vi "MFCCalAssistant.vi"() -> ()   [LabVIEW 2016]
doc: "Use this template to build a simple state machine design pattern. Each state executes code and determines which state to transition to."
uses:
  MFCCallAssistant-State.ctl
  MFCCalAssistant-Data.ctl
  Anemometry Sub Vis/Globals/Preference_global.vi
panel:
  out "Pressure":dbl format="%.1fmBar"
  out "Temp":dbl format="%.1fC"
  out "Gauge":dbl(knob) scale=0.0..10.0
  in  "Cal Gas":string(combo)
  out "Flow Rate (g/min)":dbl
  out "Flow Rate (l/min)":dbl
  out "Metered Gas Volume (ft^3)":dbl
  out "Elapsed Time (s)":dbl format="%.2f"
  out "Timer On":bool caption="(Press spacebar to toggle timer.)"
  in  "Reset Button":bool
  in  "Exit":bool
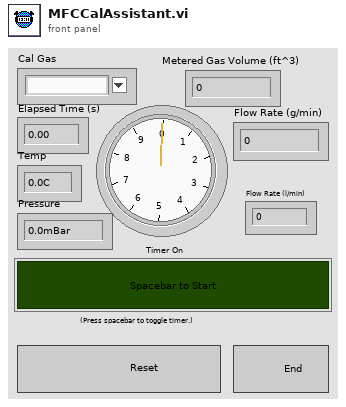
[diagram p1: front panel]
types:
  T1 = typedef "MFCCalAssistant-Data.ctl" = cluster{"Timer on?":bool, "Start Time":dbl, "Stop Time":dbl, "Elapsed Time (s)":dbl, "Measured Gas Volume (ft^3)":dbl, "Converted Gas Volume (l)":dbl, "Flow Rate (l/min)":dbl, "Flow Rate (g/min)":dbl}
  T2 = typedef "MFCCallAssistant-State.ctl" = enum16{"Initialize", "Wait for Event", "Toggle Timer", "Get User Data", "Compute Results", "Display Results", "Exit"}
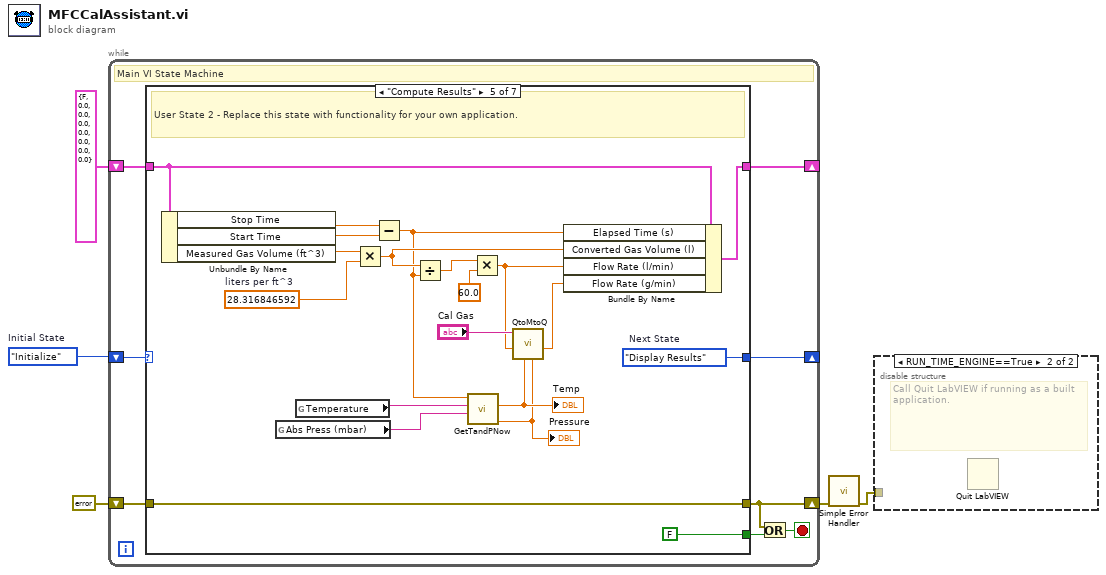
[diagram p0: block diagram]
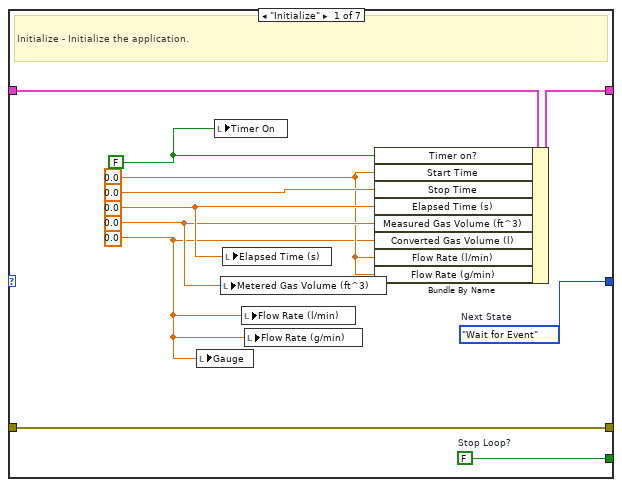
[diagram p3: hidden frame]
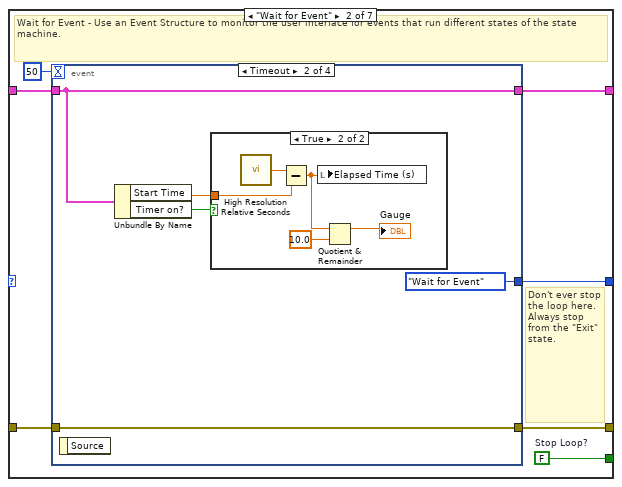
[diagram p4: hidden frame]
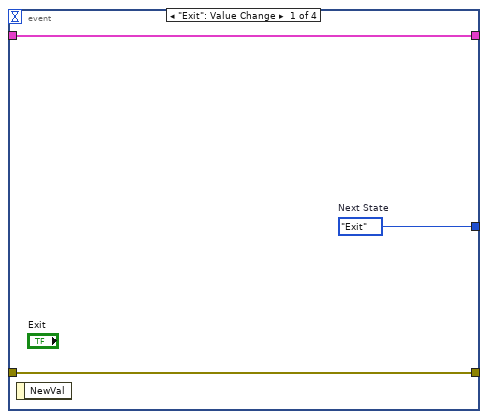
[diagram p5: hidden frame]
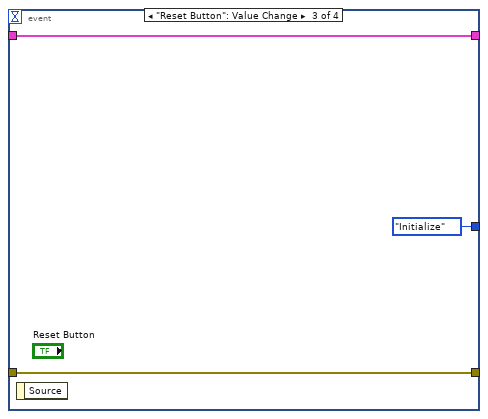
[diagram p7: hidden frame]
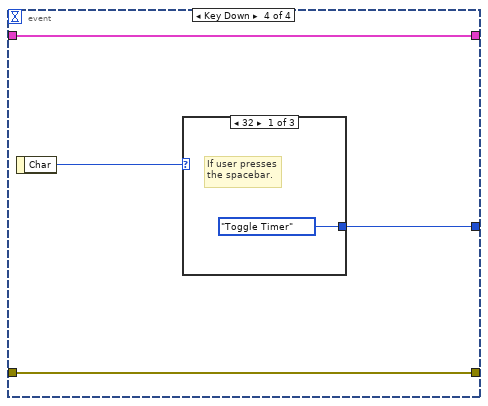
[diagram p8: hidden frame]
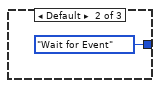
[diagram p9: hidden frame]
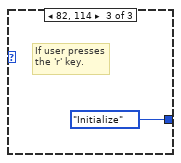
[diagram p10: hidden frame]
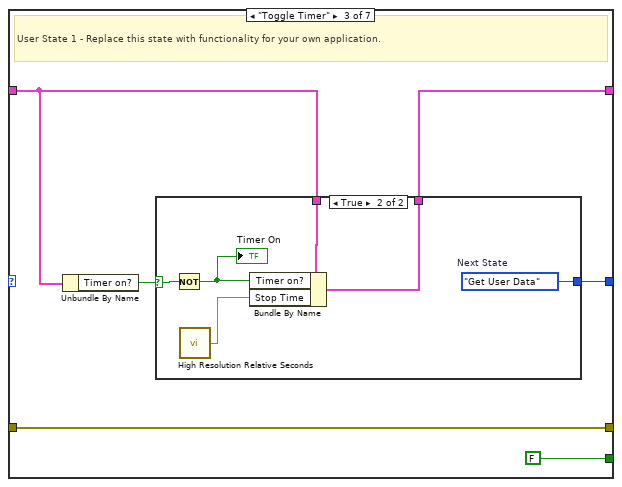
[diagram p11: hidden frame]
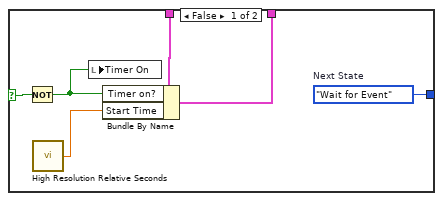
[diagram p12: hidden frame]
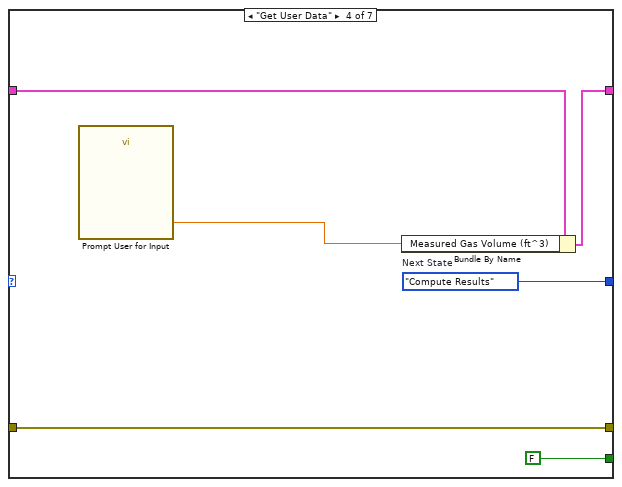
[diagram p13: hidden frame]
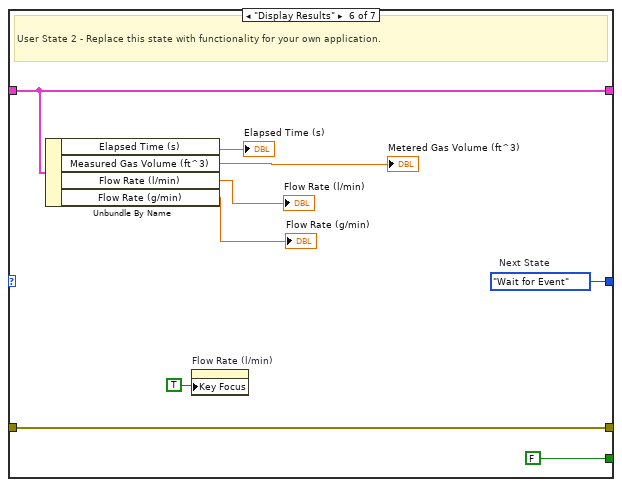
[diagram p14: hidden frame]
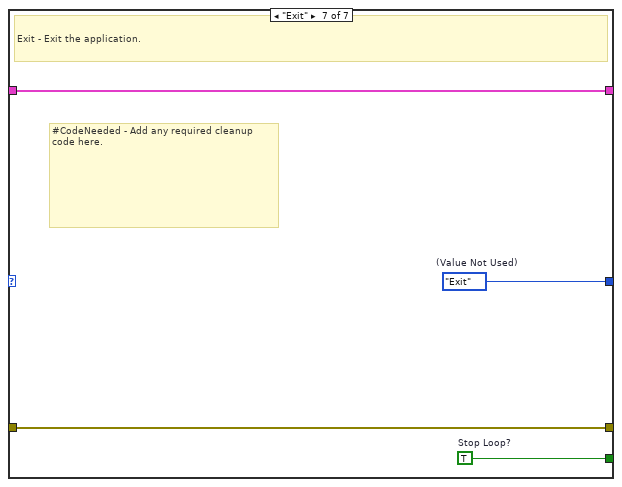
[diagram p15: hidden frame]
diagram:
  w5 = MFCCallAssistant-State."Initialize"  # Initial State
  n1 = while {
    shift-right: [w12] -> _
    shift-left: w5 -> [w13]
    shift-right: [w10] -> _
    shift-left: T1 {"Timer on?"=FALSE, "Start Time"=0.0, "Stop Time"=0.0, "Elapsed Time (s)"=0.0, "Measured Gas Volume (ft^3)"=0.0, "Converted Gas Volume (l)"=0.0, "Flow Rate (l/min)"=0.0, "Flow Rate (g/min)"=0.0} ("Data") -> [w11]
    shift-right: [w6] -> w2
    shift-left: errorcluster {"status"=FALSE, "code"=0, "source"=""} ("error constant") -> [w9]
    stop <- w7 stop-if-true
    # "Main VI State Machine"
    n2 = case shown="\"Compute Results\"" w13 {
      tunnel: [w24 w31 w57 w74 w98 w107 w111] -> w12
      tunnel: [w23 w30 FALSE ("Stop Loop?") FALSE ("Stop Loop?") FALSE ("Stop Loop?") FALSE ("Stop Loop?") w109] -> w8
      tunnel: w11 -> [w22 w29 w56 w77 w94 w104 w110]
      tunnel: [w21 w28 w55 w75 w93 w104 w110] -> w10
      tunnel: w9 -> [w20 w27 w59 w78 w96 w105 w108]
      tunnel: [w20 w26 w59 w78 w96 w105 w108] -> w6
      frame "Initialize" {
        w14 = 0.0 ("Converted Gas Volume")
        w16 = 0.0 ("Integrated Gas Volume")
        w17 = 0.0 ("Elapsed Time")
        w15 = 0.0 ("Stop Time")
        w18 = FALSE ("Replace_Me_Boolean")
        w23 = FALSE  # Stop Loop?
        w24 = MFCCallAssistant-State."Wait for Event"  # Next State
        # "Initialize - Initialize the application."
        n3 = local write "Gauge"(w14) -> ()
        n4 = local write "Timer On"(w18) -> ()
        n5 = local write "Metered Gas Volume (ft^3)"(w16) -> ()
        n6 = local write "Elapsed Time (s)"(w17) -> ()
        n7 = local write "Flow Rate (l/min)"(w14) -> ()
        n8 = local write "Flow Rate (g/min)"(w14) -> ()
        n9 = Bundle By Name(cluster=w22, "Timer on?"=w18, "Start Time"=w15, "Stop Time"=0.0 ("Start Time"), "Elapsed Time (s)"=w17, "Measured Gas Volume (ft^3)"=w16, "Converted Gas Volume (l)"=w14, "Flow Rate (l/min)"=w15, "Flow Rate (g/min)"=w15) -> (w21:T1)
      }
      frame "Wait for Event" {
        w30 = FALSE  # Stop Loop?
        # "Don't ever stop the loop here. Always stop from the \"Exit\" state."
        # "Wait for Event - Use an Event Structure to monitor the user interface for events that run different states of the state machine."
        n10 = event shown="[1] Timeout" {
          selector: _ -> [_ _ _ _]
          dyn-events: _ -> [_ _ _ _]
          timeout: 50 -> [_ _ _ _]
          tunnel: [w34 MFCCallAssistant-State."Wait for Event" ("Next State") MFCCallAssistant-State."Initialize" ("Next State") w48] -> w31
          tunnel: w29 -> [w33 w36 w47 w51]
          tunnel: [w33 w36 w47 w51] -> w28
          tunnel: w27 -> [w32 w39 w46 w50]
          tunnel: [w32 w39 w46 w50] -> w26
          event "Exit": Value Change {
            w34 = MFCCallAssistant-State."Exit"  # Next State
            n11 = event-data() -> ()  [unwired: 1 in, 1 out]
          }
          event Timeout {
            n12 = event-data() -> ()  [unwired: 1 in, 1 out]
            n13 = Unbundle By Name(w36) -> ("Start Time"=w37:dbl, "Timer on?"=w35:bool)
            n14 = case shown="True" w35 {
              tunnel: w37 -> [_ w43]
              frame False {
              }
              frame True {
                n15 = call <vilib>:"High Resolution Relative Seconds.vi"() -> ("relative seconds"=w44:dbl)
                n16 = Subtract(x=w44, y=w43) -> (x-y=w42:dbl)
                n17 = local write "Elapsed Time (s)"(w42) -> ()
                n18 = Quotient & Remainder(x=w42, y=10.0) -> (x-y*floor(x/y)=→"Gauge":dbl)  [unwired: 1 out]
              }
            }
          }
          event "Reset Button": Value Change {
            n19 = event-data() -> ()  [unwired: 1 in, 1 out]
          }
          event Key Down {
            n20 = event-data() -> ("Char"=w49:i16)  [unwired: 1 in]
            n21 = case shown="32" w49 {
              tunnel: [MFCCallAssistant-State."Toggle Timer" ("Next State") MFCCallAssistant-State."Wait for Event" ("Next State") MFCCallAssistant-State."Initialize" ("Next State")] -> w48
              frame 32 {
                # "If user presses\nthe spacebar."
              }
              frame Default {
              }
              frame 82, 114 {
                # "If user presses\nthe 'r' key."
              }
            }
          }
        }
      }
      frame "Toggle Timer" {
        # "User State 1 - Replace this state with functionality for your own application."
        n22 = Unbundle By Name(w56) -> ("Timer on?"=w58:bool)
        n23 = case shown="True" w58 {
          selector: w58 -> [w62 w68]
          tunnel: [w66 w72] -> w57
          tunnel: w56 -> [w64 w70]
          tunnel: [w63 w69] -> w55
          frame False {
            w66 = MFCCallAssistant-State."Wait for Event"  # Next State
            n24 = Not(x=w62) -> (.not. x?=w61:bool)
            n25 = call <vilib>:"High Resolution Relative Seconds.vi"() -> ("relative seconds"=w65:dbl)
            n26 = local write "Timer On"(w61) -> ()
            n27 = Bundle By Name(cluster=w64, "Timer on?"=w61, "Start Time"=w65) -> (w63:T1)
          }
          frame True {
            w72 = MFCCallAssistant-State."Get User Data"  # Next State
            n28 = Not(x=w68) -> (.not. x?=w67:bool)
            "Timer On" <- w67
            n29 = call <vilib>:"High Resolution Relative Seconds.vi"() -> ("relative seconds"=w71:dbl)
            n30 = Bundle By Name(cluster=w70, "Timer on?"=w67, "Stop Time"=w71) -> (w69:T1)
          }
        }
      }
      frame "Get User Data" {
        w74 = MFCCallAssistant-State."Compute Results"  # Next State
        n31 = call "Prompt User for Input"() -> ("Gas Volume"=w76:dbl)  [unwired: 17 in, 2 out]
        n32 = Bundle By Name(cluster=w77, "Measured Gas Volume (ft^3)"=w76) -> (w75:T1)
      }
      frame "Compute Results" {
        w92 = 28.316846592  # liters per ft^3
        w98 = MFCCallAssistant-State."Display Results"  # Next State
        # "User State 2 - Replace this state with functionality for your own application."
        n33 = Unbundle By Name(w94) -> ("Stop Time"=w89:dbl, "Start Time"=w95:dbl, "Measured Gas Volume (ft^3)"=w91:dbl)
        n34 = global read "Preference_global.vi" "Abs Press (mbar)"() -> (w80:string)
        n35 = global read "Preference_global.vi" "Temperature"() -> (w81:string)
        n36 = Multiply(x=w91, y=w92) -> (x*y=w90:dbl)
        n37 = Subtract(x=w89, y=w95) -> (x-y=w82:dbl)
        n38 = Divide(x=w90, y=w82) -> (x/y=w88:dbl)
        n39 = call "GetTandPNow.vi"("Pressure channel"=w80, "Temperature channel"=w81, "History (s)"=w82) -> ("Press (mBar)"=w79:dbl, "Temp (C)"=w86:dbl)  [unwired: 7 in]
        "Temp" <- w86
        "Pressure" <- w79
        n40 = Multiply(x=w88, y=60.0) -> (x*y=w83:dbl)
        n41 = call "QtoMtoQ.vi"("Pressure"=w79, "Temperature"=w86, "Q in (l/min)"=w83, "Gas"="Cal Gas") -> ("Mdot out (g/min)"=w84:dbl)  [unwired: 3 in, 2 out]
        n42 = Bundle By Name(cluster=w94, "Elapsed Time (s)"=w82, "Converted Gas Volume (l)"=w90, "Flow Rate (l/min)"=w83, "Flow Rate (g/min)"=w84) -> (w93:T1)
      }
      frame "Display Results" {
        w107 = MFCCallAssistant-State."Wait for Event"  # Next State
        # "User State 2 - Replace this state with functionality for your own application."
        n43 = Unbundle By Name(w104) -> ("Elapsed Time (s)"=→"Elapsed Time (s)":dbl, "Measured Gas Volume (ft^3)"=→"Metered Gas Volume (ft^3)":dbl, "Flow Rate (l/min)"=→"Flow Rate (l/min)":dbl, "Flow Rate (g/min)"=→"Flow Rate (g/min)":dbl)
        n44 = property on="Flow Rate (l/min)" class="DigNum (strict)"("Key Focus"=TRUE) -> ()  [unwired: 2 in, 2 out]
      }
      frame "Exit" {
        w109 = TRUE  # Stop Loop?
        w111 = MFCCallAssistant-State."Exit"  # (Value Not Used)
        # "#CodeNeeded - Add any required cleanup code here."
        # "Exit - Exit the application."
      }
    }
    n45 = Or(x=w6, y=w8) -> (x .or. y?=w7:bool)
  }
  n46 = call <vilib>:"Simple Error Handler.vi"("error in (no error)"=w2) -> ("error out"=w1:errorcluster)  [unwired: 4 in, 4 out]
  n47 = disable-structure shown="RUN_TIME_ENGINE==True" {
    disable-tunnel: w1 -> [_ _]
    frame condition #0 (active) {
    }
    frame condition #1 {
      # "Call Quit LabVIEW if running as a built application."
      n48 = Quit LabVIEW() -> ()  [unwired: 1 in]
    }
  }
